vi "SimpleDriveMotors.vi"(8 "error in (no error)":errorcluster, 9 "RightSpeed":dbl, 10 "LeftSpeed":dbl, 11 "RobotDriveDevRef In":T1={"DevStatus"={"status"=FALSE, "code"=0, "source"=""}, "Motors[]"=[], "Square Inputs"=FALSE, "Max Output"=1.0, "Isochronous"=FALSE}) -> (0 "error out":errorcluster, 3 "RobotDriveDevRef Out":T1={"DevStatus"={"status"=FALSE, "code"=0, "source"=""}, "Motors[]"=[], "Square Inputs"=FALSE, "Max Output"=1.0, "Isochronous"=FALSE})   [LabVIEW 2011]
uses:
  <vilib>/Rock Robotics/WPI/RobotDrive/WPI_RobotDriveDevRef.ctl
  <vilib>/Rock Robotics/WPI/MotorControl/WPI_MotorControlDeviceRef.ctl
  <vilib>/Rock Robotics/SystemInterfaces/Typedef/FPGA_TypedefDigitalModule.ctl
  <vilib>/Rock Robotics/SystemInterfaces/DIO/FPGA_DIOPWMChannel.ctl
  <vilib>/Rock Robotics/WPI/PWM/WPI_PWMDeadband.ctl
  <vilib>/Rock Robotics/WPI/CAN/Jaguar/SubVIs/WPI_CANJaguar_ControlMode.ctl
  <vilib>/Rock Robotics/WPI/PWM/WPI_PWMTransform_ConPane.ctl
  <vilib>/Rock Robotics/WPI/RobotDrive/WPI_RobotDriveMotorSelectorEnum.ctl
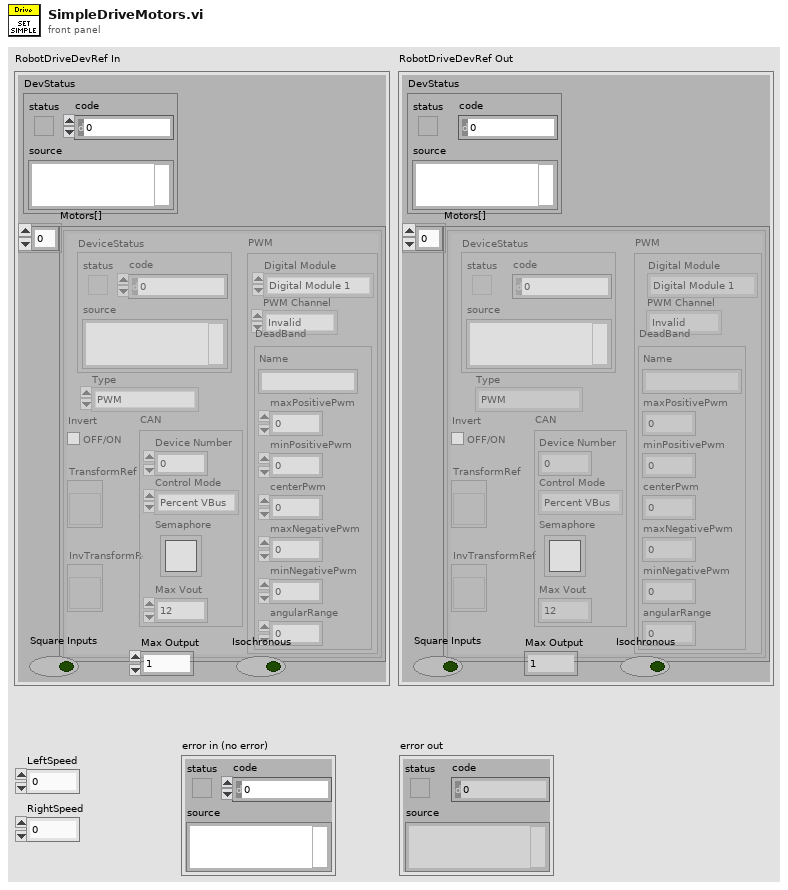
[diagram p1: front panel]
types:
  T1 = typedef "WPI_RobotDriveDevRef.ctl" = cluster{"DevStatus":errorcluster, "Motors[]":T2[], "Square Inputs":bool, "Max Output":dbl, "Isochronous":bool}
  T2 = typedef "WPI_MotorControlDeviceRef.ctl" = cluster{"DeviceStatus":errorcluster, "Type":enum16{"PWM", "CAN"}, "PWM":cluster{"Digital Module":T3, "PWM Channel":T4, "DeadBand":T5}, "CAN":cluster{"Device Number":u8, "Control Mode":T6, "Semaphore":T7, "Max Vout":dbl}, "Invert":bool, "TransformRef":T8, "InvTransformRef":T8}
  T3 = typedef "FPGA_TypedefDigitalModule.ctl" = enum16{"Digital Module 1", "Digital Module 2"}
  T4 = typedef "FPGA_DIOPWMChannel.ctl" = enum8{"PWM 1", "PWM 2", "PWM 3", "PWM 4", "PWM 5", "PWM 6", "PWM 7", "PWM 8", "PWM 9", "PWM 10", "Invalid"}
  T5 = typedef "WPI_PWMDeadband.ctl" = cluster{"Name":string, "maxPositivePwm":i32, "minPositivePwm":i32, "centerPwm":i32, "maxNegativePwm":i32, "minNegativePwm":i32, "angularRange":u16}
  T6 = typedef "WPI_CANJaguar_ControlMode.ctl" = enum8{"Percent VBus", "Current", "Speed", "Position", "Voltage"}
  T7 = typedef "Semaphore RefNum" = refnum<k1>
  T8 = typedef "WPI_PWMTransform_ConPane.ctl" = refnum<vi>
  T9 = typedef "WPI_RobotDriveMotorSelectorEnum.ctl" = enum16{"Rear Left Motor", "Rear Right Motor", "Front Left Motor", "Front Right Motor"}
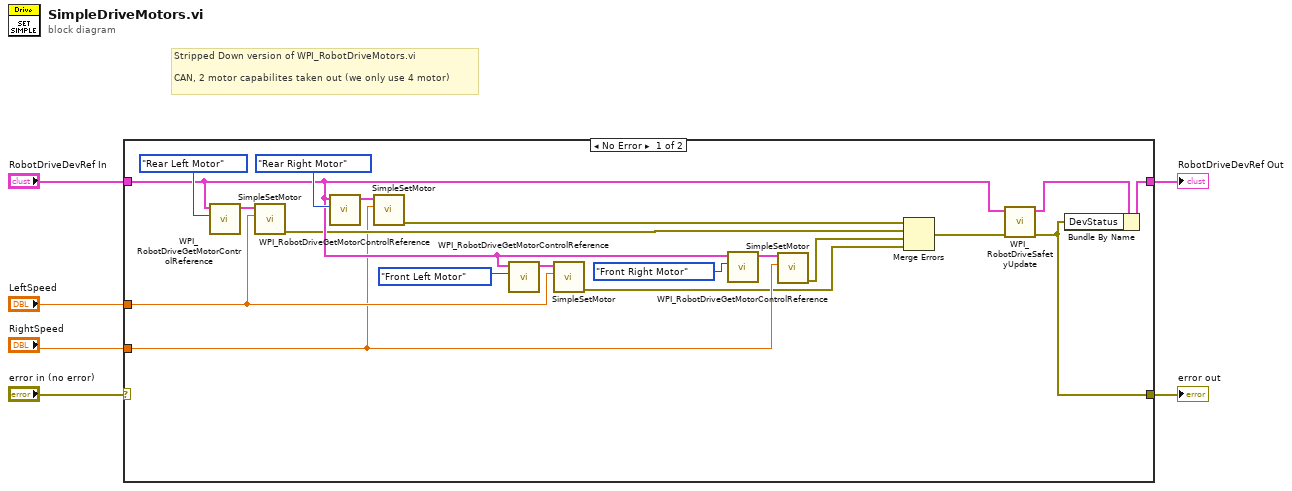
[diagram p0: block diagram]
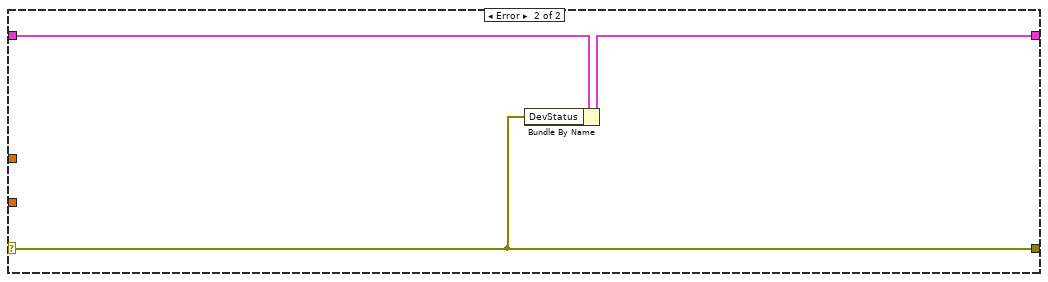
[diagram p2: hidden frame]
diagram:
  # "Stripped Down version of WPI_RobotDriveMotors.vi\n\nCAN, 2 motor capabilites taken out (we only use 4 motor)"
  n1 = case shown="No Error" "error in (no error)" {
    selector: "error in (no error)" -> [_ w27]
    tunnel: "RobotDriveDevRef In" -> [w21 w28]
    tunnel: [w18 w26] -> w5
    tunnel: "LeftSpeed" -> [w15 _]
    tunnel: "RightSpeed" -> [w9 _]
    tunnel: [w19 w27] -> w1
    frame No Error {
      n2 = call <vilib>:"WPI_RobotDriveGetMotorControlReference.vi"("MotorIndex"=WPI_RobotDriveMotorSelectorEnum."Rear Left Motor", "RobotDriveDevRef"=w21) -> ("MotorControlDeviceRef"=w16:T2)  [unwired: 9 out]
      n3 = call "SimpleSetMotor.vi"("Output"=w15, "MotorControlDevRef"=w16) -> ("error out"=w11:errorcluster)  [unwired: 8 in, 1 out]
      n4 = call <vilib>:"WPI_RobotDriveGetMotorControlReference.vi"("MotorIndex"=WPI_RobotDriveMotorSelectorEnum."Rear Right Motor", "RobotDriveDevRef"=w21) -> ("MotorControlDeviceRef"=w14:T2)  [unwired: 9 out]
      n5 = call "SimpleSetMotor.vi"("Output"=w9, "MotorControlDevRef"=w14) -> ("error out"=w12:errorcluster)  [unwired: 8 in, 1 out]
      n6 = call <vilib>:"WPI_RobotDriveGetMotorControlReference.vi"("MotorIndex"=WPI_RobotDriveMotorSelectorEnum."Front Left Motor", "RobotDriveDevRef"=w21) -> ("MotorControlDeviceRef"=w13:T2)  [unwired: 9 out]
      n7 = call "SimpleSetMotor.vi"("Output"=w15, "MotorControlDevRef"=w13) -> ("error out"=w7:errorcluster)  [unwired: 8 in, 1 out]
      n8 = call <vilib>:"WPI_RobotDriveGetMotorControlReference.vi"("MotorIndex"=WPI_RobotDriveMotorSelectorEnum."Front Right Motor", "RobotDriveDevRef"=w21) -> ("MotorControlDeviceRef"=w10:T2)  [unwired: 9 out]
      n9 = call "SimpleSetMotor.vi"("Output"=w9, "MotorControlDevRef"=w10) -> ("error out"=w8:errorcluster)  [unwired: 8 in, 1 out]
      n10 = Merge Errors(w12, w11, w8, w7) -> (w17:errorcluster)
      n11 = call <vilib>:"WPI_RobotDriveSafetyUpdate.vi"("error in (no error)"=w17, "RobotDriveDevRef"=w21) -> ("error out"=w19:errorcluster, "RobotDriveDevRef"=w20:T1)  [unwired: 8 out]
      n12 = Bundle By Name(cluster=w20, "DevStatus"=w19) -> (w18:T1)
    }
    frame Error {
      n13 = Bundle By Name(cluster=w28, "DevStatus"=w27) -> (w26:T1)
    }
  }
  "RobotDriveDevRef Out" <- w5
  "error out" <- w1
